vi "CMD_MOVENAME.vi"(6 "Gantry in":refnum<class "Gantry.lvclass">, 8 "error in (no error)":errorcluster, 10 "Arguments":string[](array[string]), 11 "gScript Interpreter in":refnum<class "gScript Interpreter.lvclass">) -> (0 "error out":errorcluster, 3 "gScript Interpreter out":refnum<class "gScript Interpreter.lvclass">, 4 "Gantry out":refnum<class "Gantry.lvclass">)   [LabVIEW 2017, in "gScript Interpreter.lvclass"]
uses:
  gScript Interpreter.lvclass
  Shared Components/Gantry Class/Gantry.lvclass
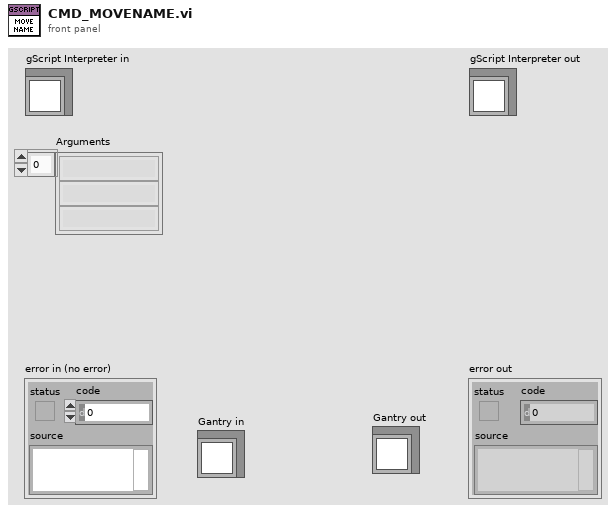
[diagram p1: front panel]
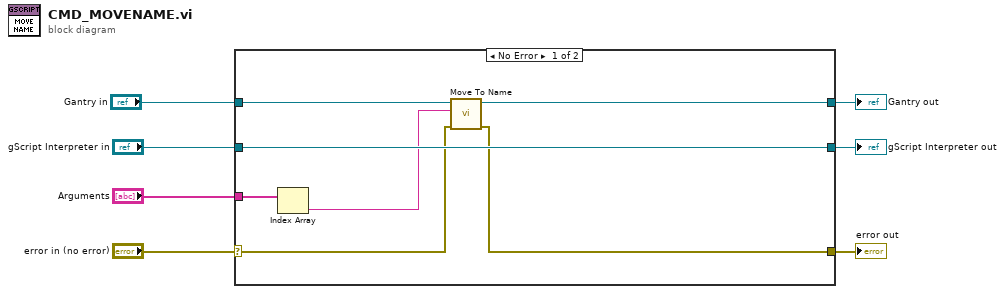
[diagram p0: block diagram]
diagram:
  n1 = case shown="No Error" "error in (no error)" {
    selector: "error in (no error)" -> [w8 w17]
    tunnel: [w10 w17] -> w6
    tunnel: [w11 w16] -> w4
    tunnel: "gScript Interpreter in" -> [w11 w16]
    tunnel: "Arguments" -> [w14 _]
    tunnel: "Gantry in" -> [w13 w15]
    tunnel: [w12 w15] -> w1
    frame No Error {
      n2 = Index Array(array=w14) -> (element=w9:string)  [unwired: 1 in]
      n3 = call-dynamic "Move To Name.vi"("error in"=w8, "Destination"=w9, "Gantry in"=w13) -> ("error out"=w10:errorcluster, "Gantry out"=w12:refnum<class "Gantry.lvclass">)  [unwired: 7 in]
    }
    frame Error {
    }
  }
  "error out" <- w6
  "gScript Interpreter out" <- w4
  "Gantry out" <- w1
